vi "GT Get Soft Limit.vi"(7 "pNegative":i32, 8 "error in (no error)":errorcluster caption="错误输入（无错误）", 9 "pPositive":i32, 10 "axis":i16, 11 "cardNum":i16) -> (0 "error out":errorcluster caption="错误输出", 1 "pPositive out":i32, 3 "function return":i16, 5 "pNegative out":i32)   [LabVIEW 2020, in "gts.lvlib"]
doc: "GT_API GT_GetSoftLimit(short cardNum,short axis,long *pPositive,long *pNegative);"
uses:
  gts.lvlib
  dll/32bit/multi_card/gts.dll
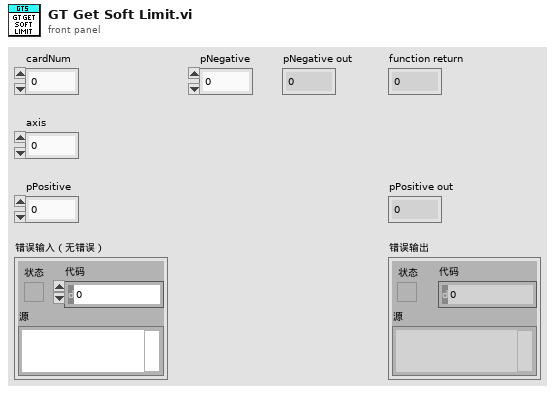
[diagram p1: front panel]
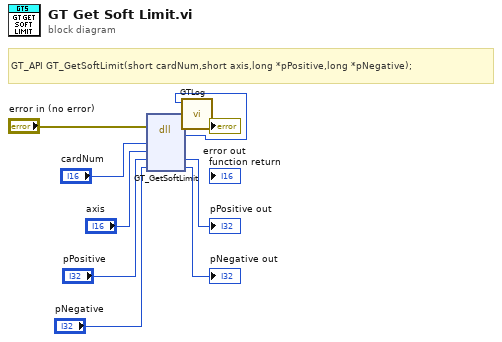
[diagram p0: block diagram]
diagram:
  # "GT_API GT_GetSoftLimit(short cardNum,short axis,long *pPositive,long *pNegative);"
  n1 = dll-call lib="C:/1228/dll/32bit/multi_card/gts.dll" fn="GT_GetSoftLimit"(error in="error in (no error)", "cardNum"="cardNum", "axis"="axis", "pPositive"="pPositive", "pNegative"="pNegative") -> (error out=w3:errorcluster, w1:i16, "pPositive"=→"pPositive out":i32, "pNegative"=→"pNegative out":i32)  [unwired: 4 in, 1 out]
  n2 = call "GTLog.vi"("error in (no error)"=w3, "Numeric"=w1) -> ("error out"=→"error out":errorcluster)  [unwired: 9 in]
